vi "Label Waveform.vi"(5 "Unique Channel Name":string, 7 "Measurement":string, 11 "Input waveform":waveform(dbl)) -> (3 "Labelled Waveform":waveform(dbl))   [LabVIEW 2023, in "Instruments.lvlib" / "Instruments.lvclass"]
uses:
  Library/Instruments.lvclass
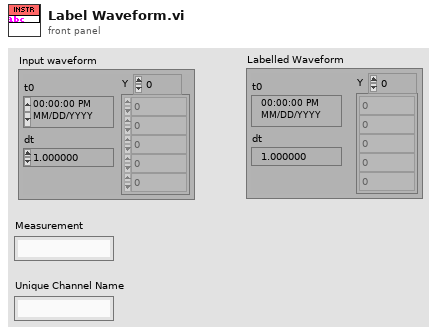
[diagram p1: front panel]
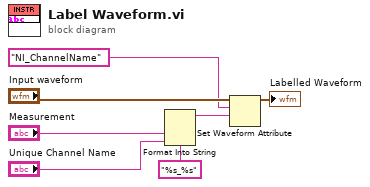
[diagram p0: block diagram]
diagram:
  n1 = Format Into String(format string="%s_%s", "Measurement", "Unique Channel Name") -> (resulting string=w3:string)  [unwired: 2 in, 1 out]
  n2 = Set Waveform Attribute(5:w3, 6:"NI_ChannelName" ("name"), 7:"Input waveform") -> (3:→"Labelled Waveform":waveform(dbl))  [unwired: 1 in, 2 out]
